vi "Generate Test Case.vi"(8 "error in (no error)":errorcluster, 11 "Process Generator In":refnum<class "Process Generator.lvclass">) -> (0 "error out":errorcluster, 3 "Process Generator Out":refnum<class "Process Generator.lvclass">)   [LabVIEW 2020, in "Process Generator.lvclass"]
uses:
  Process Generator.lvclass
  Process Generator.lvclass/Process Generator.ctl
  <vilib>/Utility/traverseref.llb/TRef TravTarget.ctl
  <vilib>/Utility/traverseref.llb/VI Scripting - Traverse.lvlib
  <vilib>/Asteme/LUnit/Test Case.lvclass
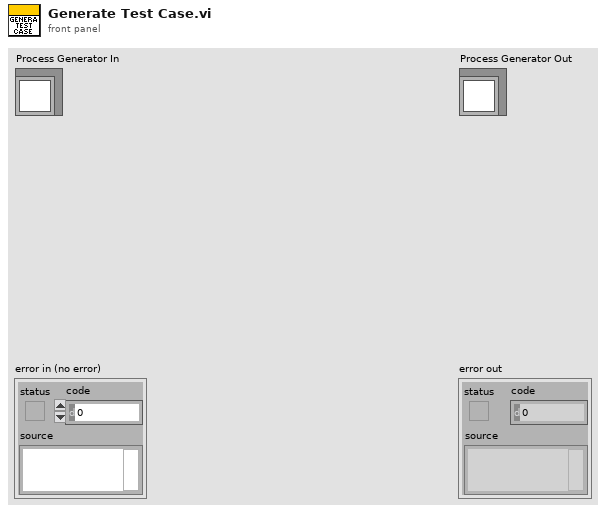
[diagram p1: front panel]
types:
  T1 = typedef "TRef TravTarget.ctl" = enum16{"FP", "BD", "Other"}
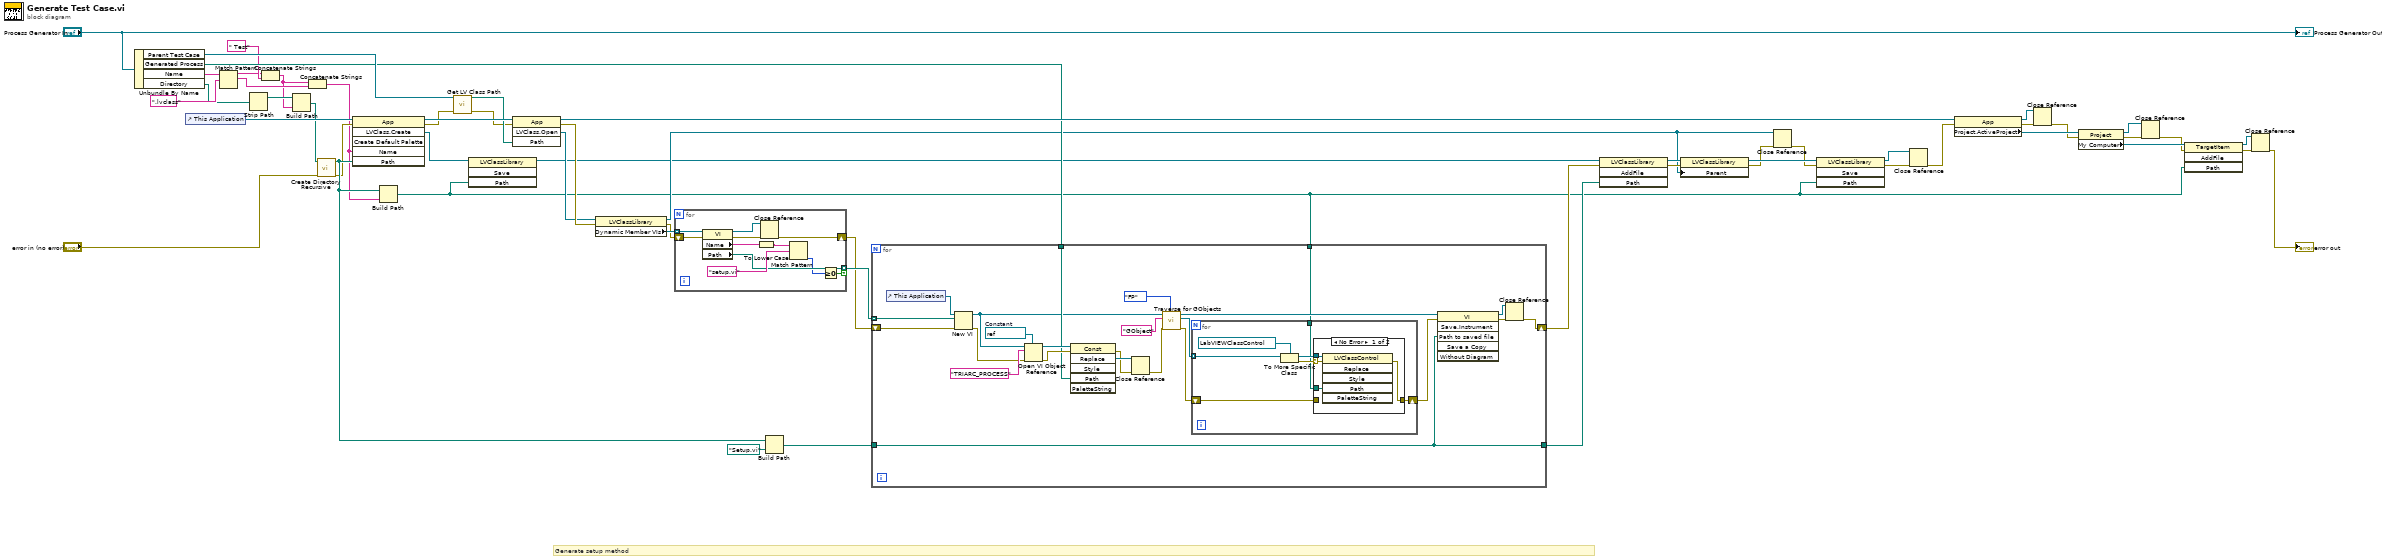
[diagram p0: block diagram]
diagram:
  # "Generate setup method"
  n1 = Unbundle By Name("Process Generator In") -> ("Parent Test Case"=w54:refnum<class "Test Case.lvclass">, "Generated Process"=w30:path, "Name"=w10:string, "Directory"=w6:path)
  n2 = control-ref of="This Application"() -> (w23:refnum<vi>)
  n3 = Match Pattern(string=w10, regular expression=".lvclass" ("string")) -> (before substring=w7:string, match substring=w4:string)  [unwired: 1 in, 2 out]
  n4 = Strip Path(path=w6) -> (stripped path=w3:path)  [unwired: 1 out]
  n5 = Concatenate Strings(w7, " Test" ("string")) -> (w2:string)
  n6 = Build Path(base path=w3, name or relative path=w2) -> (appended path=w1:path)
  n7 = Concatenate Strings(w2, w4) -> (w5:string)
  n8 = call <vilib>:"Create Directory Recursive.vi"("error in (no error)"="error in (no error)", "directory"=w1) -> ("error out"=w24:errorcluster, "directory copy"=w28:path)  [unwired: 3 in, 1 out]
  n9 = invoke class="App" method="LVClass.Create"(reference=w23, error in=w24, "Name"=w5, "Path"=w28) -> (reference out=w53:refnum<vi>, error out=w42:errorcluster, "LVClass.Create"=w13:refnum<vi>)  [unwired: 2 in, 3 out]
  n10 = Build Path(base path=w28, name or relative path=w5) -> (appended path=w11:path)
  n11 = call <vilib>:"Get LV Class Path.vi"("error in (no error)"=w42, "object"=w54) -> ("error out"=w41:errorcluster, "class path"=w52:path)  [unwired: 8 in]
  n12 = invoke class="LVClassLibrary" method="Save"(reference=w13, "Path"=w11) -> (reference out=w12:refnum<vi>)  [unwired: 2 in, 3 out]
  n13 = invoke class="App" method="LVClass.Open"(reference=w53, error in=w41, "Path"=w52) -> (reference out=w51:refnum<vi>, error out=w21:errorcluster, "LVClass.Open"=w16:refnum<vi>)  [unwired: 1 in, 1 out]
  n14 = property class="LVClassLibrary"(reference=w16, error in=w21) -> (reference out=w14:refnum<vi>, error out=w31:errorcluster, "Dynamic Member VIs"=w34:refnum<vi>[])
  n15 = for {
    tunnel: w34 -> [w66] mode=indexing
    shift-right: [w59] -> w32
    shift-left: w31 -> [w62]
    tunnel: [w60] -> w33 mode=indexing if=w57
    n16 = property class="VI"(reference=w66, error in=w62) -> (reference out=w58:refnum<vi>, error out=w61:errorcluster, "Name"=w65:string, "Path"=w60:path)
    n17 = To Lower Case(string=w65) -> (all lower case string=w64:string)
    n18 = Close Reference(reference=w58, error in (no error)=w61) -> (error out=w59:errorcluster)
    n19 = Match Pattern(string=w64, regular expression="setup.vi" ("y")) -> (offset past match=w56:i32)  [unwired: 1 in, 3 out]
    n20 = Greater Or Equal To 0?(x=w56) -> (x >= 0?=w57:bool)
  }
  n21 = Build Path(base path=w28, name or relative path=path "Setup.vi") -> (appended path=w26:path)
  n22 = for {
    tunnel: w33 -> [w90] mode=indexing
    shift-right: [w79] -> w29
    shift-left: w32 -> [w89]
    tunnel: w30 -> [w83]
    tunnel: w26 -> [w77]
    tunnel: [w77] -> w25
    tunnel: w11 -> [w70]
    w87 = refnum<vi> refnum  # Constant
    n23 = control-ref of="This Application"() -> (w67:refnum<vi>)
    n24 = New VI(8:w89, 10:w90, 11:w67) -> (0:w86:errorcluster, 3:w76:refnum<vi>)  [unwired: 4 in]
    n25 = Open VI Object Reference(7:w87, 8:w86, 10:"TRIARC_PROCESS" ("name/order"), 11:w76) -> (0:w84:errorcluster, 3:w85:refnum<vi>)
    n26 = invoke on="Invoke Node" class="Const" method="Replace"(reference=w85, error in=w84, "Path"=w83) -> (error out=w81:errorcluster, "Replace"=w82:refnum<vi>)  [unwired: 3 in, 4 out]
    n27 = Close Reference(reference=w82, error in (no error)=w81) -> (error out=w72:errorcluster)
    n28 = call <vilib>:"Traverse for GObjects.vi"("Traverse Target"=TRef_TravTarget."FP", "error in (no error)"=w72, "Class Name"="GObject", "VI Refnum"=w76) -> ("error out"=w68:errorcluster, "References"=w71:refnum<vi>[], "dup VI Refnum"=w75:refnum<vi>)  [unwired: 4 in, 1 out]
    n29 = for {
      tunnel: w71 -> [w97] mode=indexing
      tunnel: w70 -> [w93]
      shift-right: [w92] -> w69
      shift-left: w68 -> [w91]
      n30 = To More Specific Class(target class=refnum<vi> refnum ("reference out"), reference=w97) -> (specific class reference=w94:refnum<vi>, error out=w95:errorcluster)  [unwired: 1 in]
      n31 = case shown="No Error" w95 {
        selector: w95 -> [w101 _]
        tunnel: w94 -> [w100 _]
        tunnel: w93 -> [w99 _]
        tunnel: [w98 w102] -> w92
        tunnel: w91 -> [_ w102]
        frame No Error {
          n32 = invoke on="Invoke Node" class="LVClassControl" method="Replace"(reference=w100, error in=w101, "Path"=w99) -> (error out=w98:errorcluster)  [unwired: 3 in, 5 out]
        }
        frame Error {
        }
      }
    }
    n33 = invoke on="Invoke Node" class="VI" method="Save.Instrument"(reference=w75, error in=w69, "Path to saved file"=w77) -> (reference out=w78:refnum<vi>, error out=w80:errorcluster)  [unwired: 3 in, 4 out]
    n34 = Close Reference(reference=w78, error in (no error)=w80) -> (error out=w79:errorcluster)
  }
  n35 = invoke class="LVClassLibrary" method="AddFile"(reference=w12, error in=w29, "Path"=w25) -> (reference out=w20:refnum<vi>, error out=w18:errorcluster)  [unwired: 1 in, 2 out]
  n36 = property class="LVClassLibrary"(reference=w20, error in=w18, "Parent"=w14) -> (reference out=w19:refnum<vi>, error out=w17:errorcluster)
  n37 = Close Reference(reference=w14, error in (no error)=w17) -> (error out=w15:errorcluster)
  n38 = invoke class="LVClassLibrary" method="Save"(reference=w19, error in=w15, "Path"=w11) -> (reference out=w22:refnum<vi>, error out=w47:errorcluster)  [unwired: 1 in, 2 out]
  n39 = Close Reference(reference=w22, error in (no error)=w47) -> (error out=w46:errorcluster)
  n40 = property class="App"(reference=w51, error in=w46) -> (reference out=w39:refnum<vi>, error out=w49:errorcluster, "Project.ActiveProject"=w50:refnum<vi>)
  n41 = Close Reference(reference=w39, error in (no error)=w49) -> (error out=w40:errorcluster)
  n42 = property class="Project"(reference=w50, error in=w40) -> (reference out=w37:refnum<vi>, error out=w45:errorcluster, "My Computer"=w48:refnum<vi>)
  n43 = Close Reference(reference=w37, error in (no error)=w45) -> (error out=w38:errorcluster)
  n44 = invoke class="TargetItem" method="AddFile"(reference=w48, error in=w38, "Path"=w11) -> (reference out=w35:refnum<vi>, error out=w44:errorcluster)  [unwired: 1 in, 2 out]
  n45 = Close Reference(reference=w35, error in (no error)=w44) -> (error out=→"error out":errorcluster)
  "Process Generator Out" <- "Process Generator In"
